vi "Get Project Info.vi"(8 "error in (no error)":errorcluster, 11 "Fake Project Inspector in":refnum<class "Fake Project Inspector.lvclass">) -> (0 "error out":errorcluster, 1 "Path":path, 2 "Name":string, 3 "Fake Project Inspector out":refnum<class "Fake Project Inspector.lvclass">, 4 "Item Paths":path[](array[path]))   [LabVIEW 2017, in "Cobertura.Tests.lvlib" / "Fake Project Inspector.lvclass"]
uses:
  Fake Project Inspector.lvclass
  Fake Project Inspector.lvclass/Fake Project Inspector.ctl
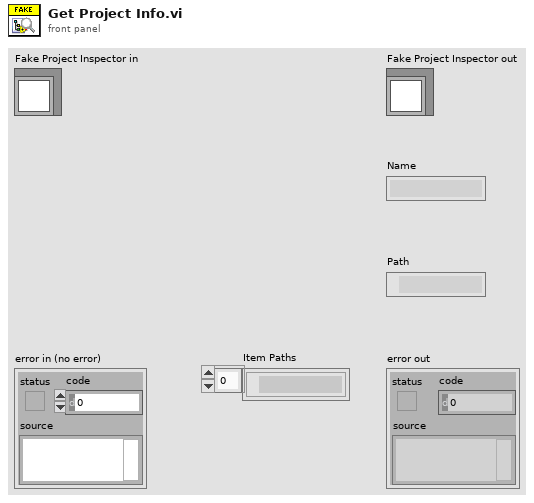
[diagram p1: front panel]
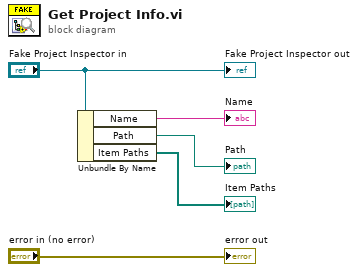
[diagram p0: block diagram]
diagram:
  n1 = Unbundle By Name("Fake Project Inspector in") -> ("Name"=→"Name":string, "Path"=→"Path":path, "Item Paths"=→"Item Paths":path[])
  "error out" <- "error in (no error)"
  "Fake Project Inspector out" <- "Fake Project Inspector in"
